vi "DDE Execute.vi"(7 "timeout (-1)":i32, 8 "error in (no error)":errorcluster, 10 "command":string, 11 "conversation refnum in":u32) -> (0 "error out":errorcluster, 3 "conversation refnum out":u32)   [LabVIEW 2018]
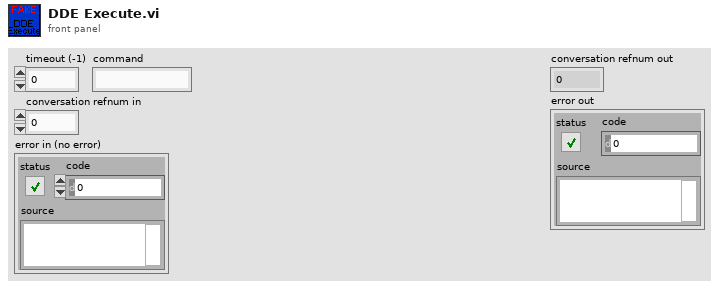
[diagram p1: front panel]
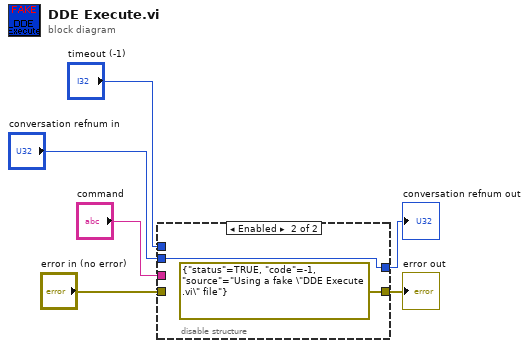
[diagram p0: block diagram]
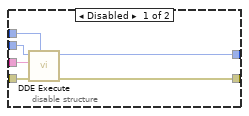
[diagram p2: hidden frame]
diagram:
  n1 = disable-structure shown="Enabled" {
    disable-tunnel: "timeout (-1)" -> [w12 _]
    disable-tunnel: "conversation refnum in" -> [w11 w13]
    disable-tunnel: "command" -> [w10 _]
    disable-tunnel: "error in (no error)" -> [w9 _]
    disable-tunnel: [w8 w13] -> w2
    disable-tunnel: [w7 errorcluster {"status"=TRUE, "code"=-1, "source"="Using a fake \"DDE Execute .vi\" file"} ("error out")] -> w1
    frame Disabled {
      n2 = call "DDE Execute.vi"("timeout (-1)"=w12, "error in (no error)"=w9, "command"=w10, "conversation refnum in"=w11) -> ("error out"=w7:errorcluster, "conversation refnum out"=w8:u32)  [unwired: 4 in]
    }
    frame Enabled {
    }
  }
  "conversation refnum out" <- w2
  "error out" <- w1
